vi "Old_Currentvstime.vi"() -> ()   [LabVIEW 2018]
uses:
  <userlib>/KE237.LLB/Keith 237 Operate/Standby.vi
  <vilib>/Utility/file.llb/Write To Spreadsheet File (string).vi
  <instrlib>/Keithley 24XX/Keithley 24XX.lvlib
  <vilib>/Analysis/NI_AALBase.lvlib
panel:
  in  "Autozero?":u16(ring)=2 items=["On", "Off", "Once"]
  in  "Measurement Speed (1 PLC)":dbl=1.0 format="%.2g"
  in  "Manual Range (Max I)":dbl=1.0
  in  "Enable Meas Auto Range":bool=TRUE
  in  "Source Mode":u16(ring) items=["Voltage", "Current"]
  in  "Measurement Gate Bias (V)":dbl=-0.85 format="%#.3g"
  in  "Initial Gate Bias (V)":dbl format="%#.3g"
  in  "Voltage Compliance Limit 237 (V)":dbl=10.0 format="%#.3f"
  in  "Current Compliance\nLimit 237 (A)":dbl=0.1 format="%#.3f"
  in  "Delay Gate (s)":dbl=60.0 format="%#.3g"
  in  "Keithley 237 GPIB address":string="17"
  in  "Wait Time Btwn Keithley Readings (ms)":i32=30
  out "Time Btwn Iterations (ms)":i32
  out "Total Elapsed Time (ms)":i32
  out "# Avgs":i32
  out "Current (A)":dbl format="%.2e"
  in  "Total Measure Time (s)":dbl=60.0 format="%#.3g"
  in  "Drain Bias (V)":dbl=-0.6 format="%#.3g"
  in  "Current Compliance\nLimit (A)":dbl=0.5 format="%#.3e"
  in  "Keithley 2400\nVISA resource":refnum<visa-resource-name>="GPIB0::24::INSTR"
  in  "Active Area (cm^2)":dbl=0.0122 min=0.0 format="%#.4e"
  in  "ApproximateTime Step (ms)":dbl=300.0 format="%#.3g"
  in  "Show Current:":enum32{"Density (mA/cm^2)", "Absolute (A)"}(radio)=enum."Absolute (A)"
  in  "Current Offset":dbl format="%^#_3e"
  out "I-t Measurement\nBy M. Ziffer 7/3/2014":cluster{dbl[], dbl[]}(graph)={[-2.0, -1.95, -1.9, -1.85, -1.8, -1.75, -1.7, -1.65, -1.6, -1.55, -1.5, -1.45, -1.4, -1.35, -1.2999999999999998, -1.25, -1.2, -1.15, -1.1, -1.0499999999999998, -1.0, -0.95, -0.8999999999999999, -0.8499999999999999, -0.7999999999999998, -0.75, -0.7, -0.6499999999999999, -0.5999999999999999, -0.5499999999999998, -0.5, -0.44999999999999996, -0.3999999999999999, -0.34999999999999987, -0.2999999999999998, -0.25, -0.19999999999999996, -0.1499999999999999, -0.09999999999999987, -0.04999999999999982, 0.0, 0.050000000000000266, 0.10000000000000009, 0.1499999999999999, 0.20000000000000018, 0.25, 0.30000000000000027, 0.3500000000000001, 0.40000000000000036, 0.4500000000000002, 0.5, 0.5500000000000003, 0.6000000000000001, 0.6500000000000004, 0.7000000000000002, 0.75, 0.8000000000000003, 0.8500000000000001, 0.9000000000000004, 0.9500000000000002, 1.0, 1.0500000000000003, 1.1, 1.1500000000000004, 1.2000000000000002, 1.25, 1.3000000000000003, 1.35, 1.4000000000000004, 1.4500000000000002, 1.5, 1.5500000000000003, 1.6, 1.6500000000000004, 1.7000000000000002, 1.75, 1.8000000000000003, 1.85, 1.9000000000000004, 1.9500000000000002, 2.0, 1.95, 1.9, 1.85, 1.8, 1.75, 1.7, 1.65, 1.6, 1.55, 1.5, 1.45, 1.4, 1.35, 1.2999999999999998, 1.25, 1.2, 1.15, 1.1, 1.0499999999999998, 1.0, 0.95, 0.8999999999999999, 0.8499999999999999, 0.7999999999999998, 0.75, 0.7, 0.6499999999999999, 0.5999999999999999, 0.5499999999999998, 0.5, 0.44999999999999996, 0.3999999999999999, 0.34999999999999987, 0.2999999999999998, 0.25, 0.19999999999999996, 0.1499999999999999, 0.09999999999999987, 0.04999999999999982, 0.0, -0.050000000000000266, -0.10000000000000009, -0.1499999999999999, -0.20000000000000018, -0.25, -0.30000000000000027, -0.3500000000000001, -0.40000000000000036, -0.4500000000000002, -0.5, -0.5500000000000003, -0.6000000000000001, -0.6500000000000004, -0.7000000000000002, -0.75, -0.8000000000000003, -0.8500000000000001, -0.9000000000000004, -0.9500000000000002, -1.0, -1.0500000000000003, -1.1, -1.1500000000000004, -1.2000000000000002, -1.25, -1.3000000000000003, -1.35, -1.4000000000000004, -1.4500000000000002, -1.5, -1.5500000000000003, -1.6, -1.6500000000000004, -1.7000000000000002, -1.75, -1.8000000000000003, -1.85, -1.9000000000000004, -1.9500000000000002, -2.0], [-0.9617289445307117, -0.9618513744908972, -0.9601574911889584, -0.9603488957746004, -0.9598860982876659, -0.9595594700613103, -0.9590290885663679, -0.9586886097902229, -0.9580144940757807, -0.9570474587019399, -0.9571418538143588, -0.9562287187728303, -0.9551771894828052, -0.9535572870291384, -0.9535421571112963, -0.9533114258642045, -0.9520938012261039, -0.9513117179729429, -0.9508812384355169, -0.9504840780921618, -0.9504173840793213, -0.9482281628421478, -0.9464640811713977, -0.9453356785488072, -0.9439408336230415, -0.9428695575652444, -0.9416178906119992, -0.9396031084275935, -0.9378375248899987, -0.9354517815949719, -0.9324159524550173, -0.928767917889437, -0.9245502864168607, -0.9203528467096396, -0.9146985405384399, -0.908595454304189, -0.9012966039381313, -0.8917361646028689, -0.8808115851751085, -0.8684870433493713, -0.853007079283089, -0.8360736418594031, -0.8154860511533626, -0.7920970894092216, -0.7641180332150388, -0.7294003786125389, -0.6854183749419586, -0.6263231964633708, -0.5399961516707377, -0.4044042921440459, -0.19129744134883978, 0.11936942255465804, 0.5420583260977958, 1.0996962734707192, 1.8318907919106253, 2.7834859177196174, 3.9948214605959804, 5.494887344369723, 7.293988211209965, 9.39251059714275, 11.765998658717283, 14.371720946722268, 17.153138293174568, 20.070768287470067, 23.082285540692517, 26.15604905590766, 29.26009131920428, 32.38734131897913, 35.54092126952808, 38.70923397757575, 41.89103456238207, 45.09512285116253, 48.318234786641504, 51.57411300669423, 54.84161623237131, 58.130390342544004, 61.4596508891188, 64.79419021952893, 68.17503711098149, 71.57587551887687, 75.0023346626475, 71.8977923333163, 68.72637799211101, 65.51757272894447, 62.2950059155054, 59.076872390492845, 55.84672949319313, 52.615591470047114, 49.383497814590335, 46.15858586388574, 42.93308596012382, 39.714879010509975, 36.494540522470736, 33.276879251143754, 30.087779593472593, 26.903443634933772, 23.758388169345494, 20.669969771208738, 17.671195580039395, 14.804861569698371, 12.12778391916459, 9.68736655227705, 7.528128139792144, 5.673530623057721, 4.128839936603901, 2.8787577310032053, 1.895544581260216, 1.1383875896205915, 0.5622048852612092, 0.12746496878202787, -0.18928305409978952, -0.4042961076690051, -0.5411369085387429, -0.6286316214282486, -0.6871327837574404, -0.7298882072135505, -0.7640718647157413, -0.7921132761963248, -0.8155779431543743, -0.8358809022810104, -0.8523300154596555, -0.8668520109778625, -0.8802307520791266, -0.8907705198464766, -0.8998007445608903, -0.9078572589377096, -0.9150023626386364, -0.9215738644543149, -0.925261336930741, -0.9288795566582202, -0.9332418679701618, -0.9352489739462505, -0.9376688708058178, -0.9394550911063516, -0.9405290371496502, -0.9430050037047499, -0.9440335043698243, -0.9453382929096107, -0.9473152502994113, -0.9474565926568992, -0.9494901203645137, -0.94896546821346, -0.9503187058651598, -0.9511280452203158, -0.9523093469306558, -0.9532668704811476, -0.9541692143312739, -0.9545545822386634, -0.955485183435348, -0.9561708134622656, -0.956805602515258, -0.9577699122788996, -0.9578049002139094, -0.9580356870856992, -0.958780001168953, -0.9592832934359943, -0.9588639388381576, -0.959203916992021, -0.9603773199952523, -0.9611007191920772, -0.9623172869609168]}
  in  "First bias settle (ms)":dbl=2000.0 format="%#.2f"
  out "Outputfile":path
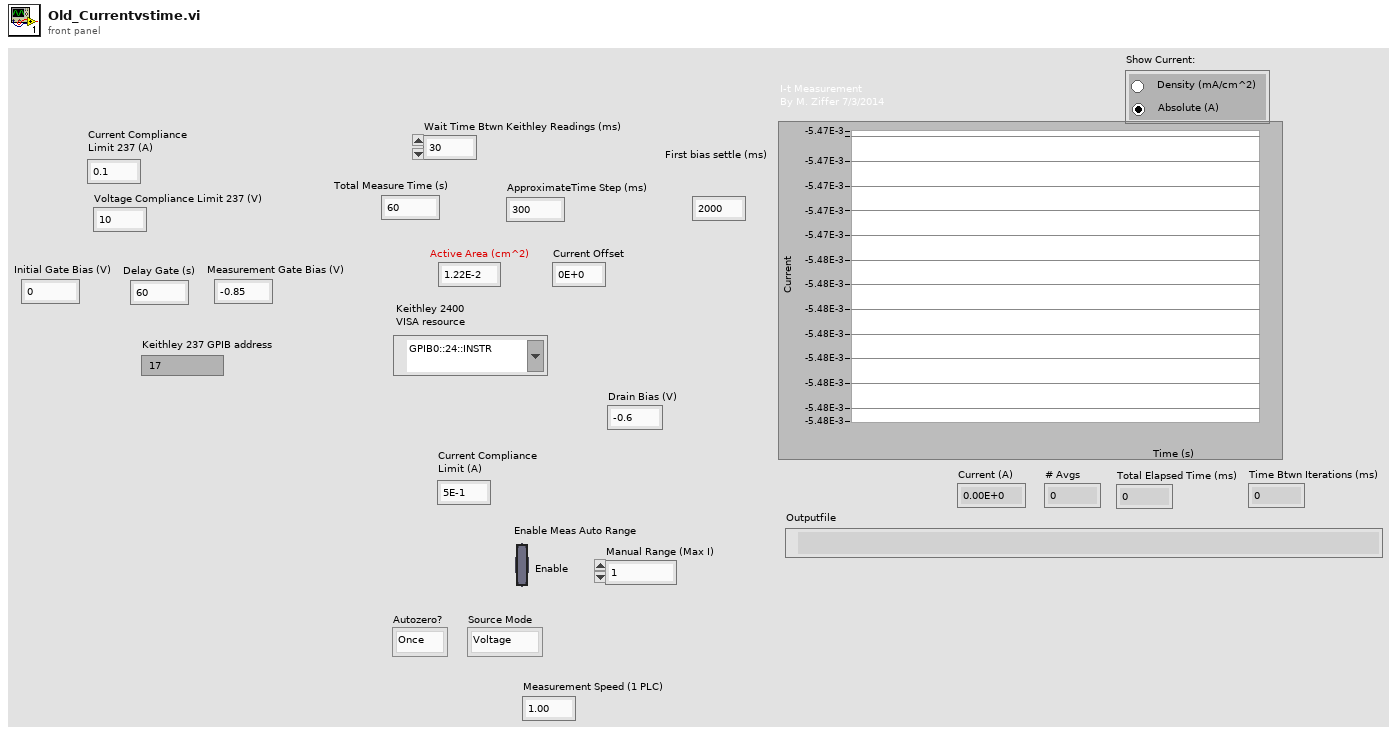
[diagram p1: front panel]
types:
  T1 = cluster{"error":bool, "code":i32, "source":string}
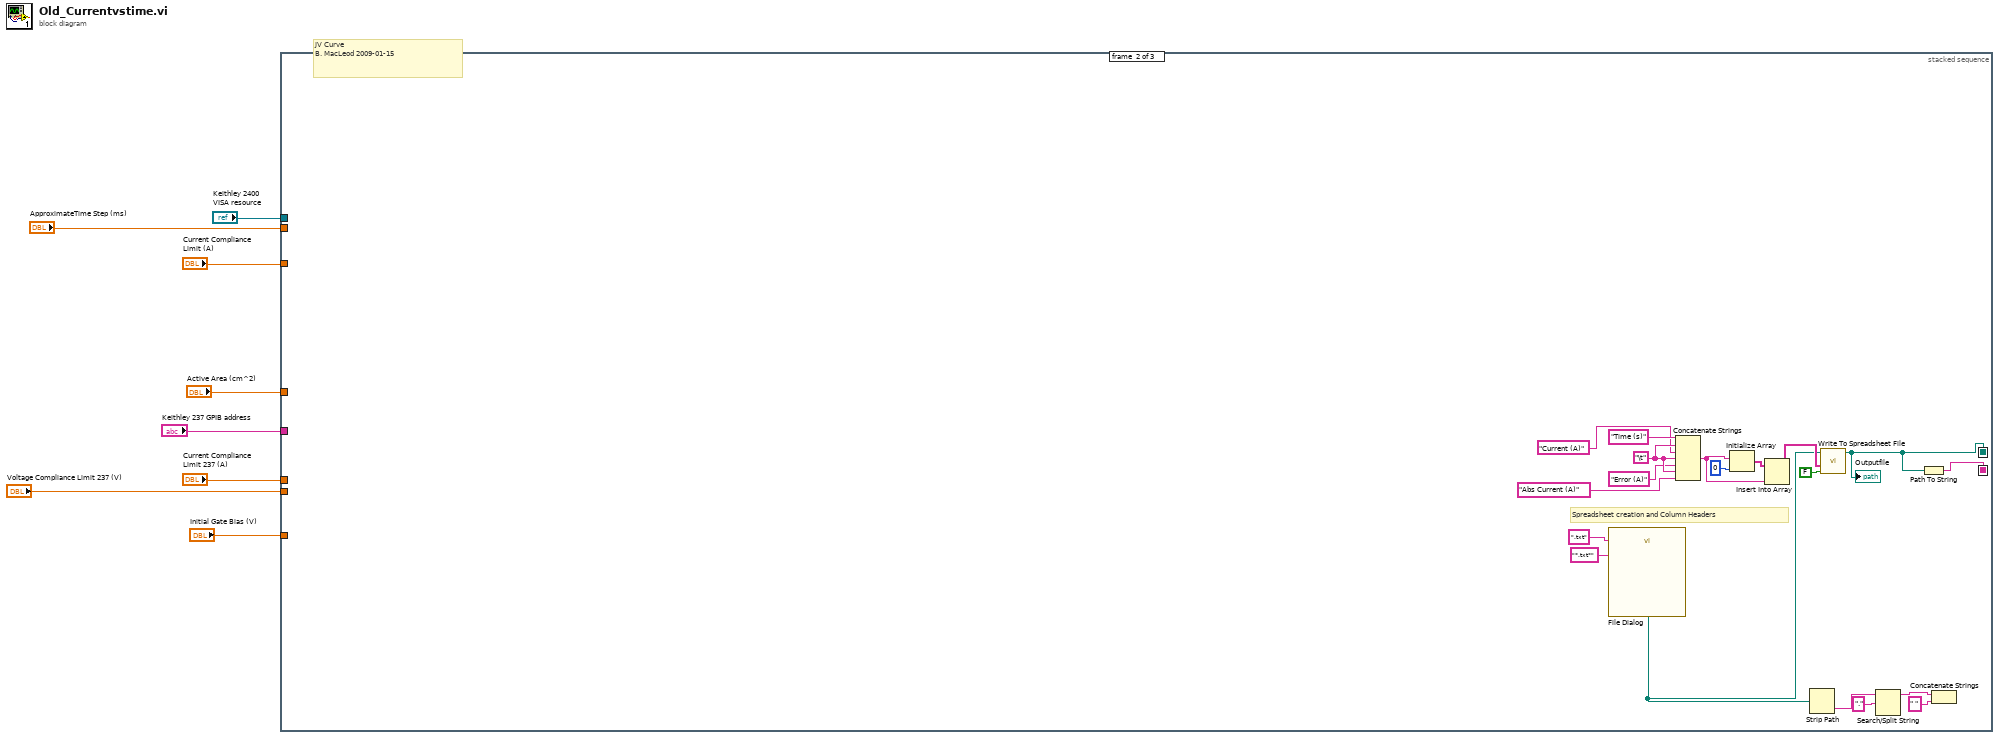
[diagram p0: block diagram]
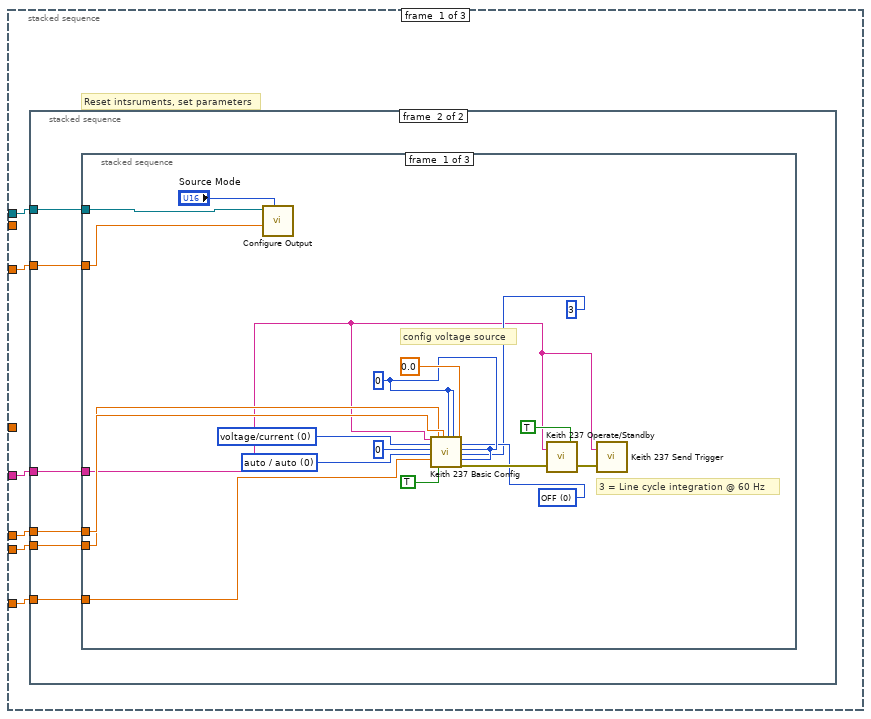
[diagram p2: hidden frame]
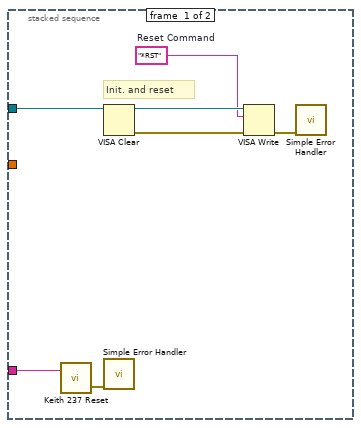
[diagram p3: hidden frame]
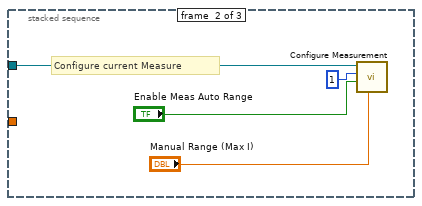
[diagram p4: hidden frame]
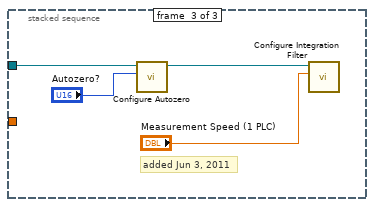
[diagram p5: hidden frame]
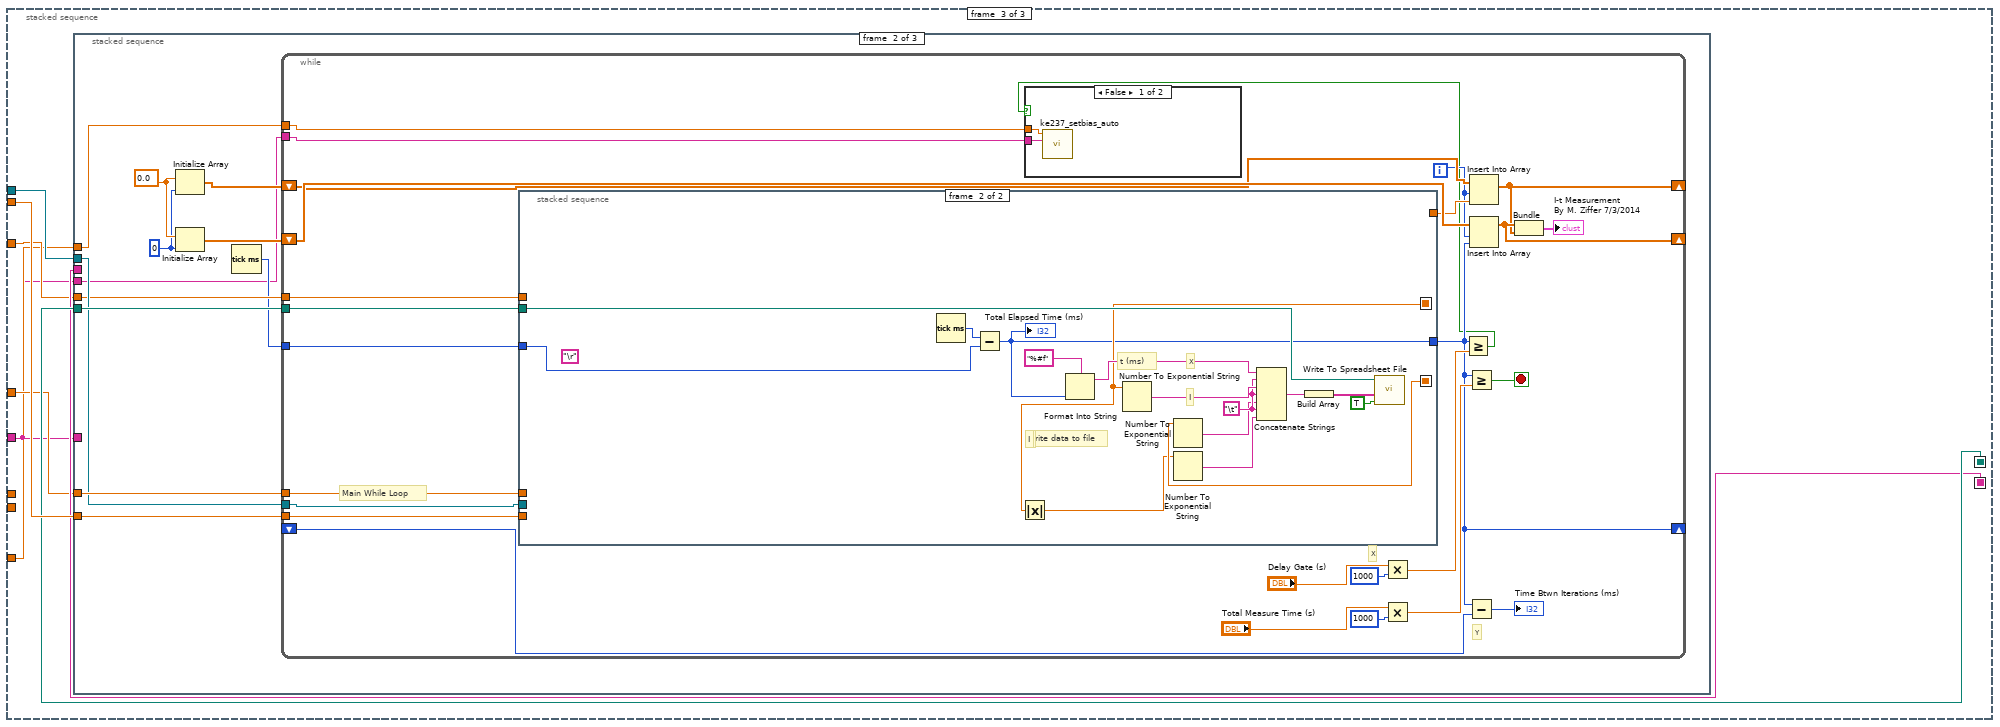
[diagram p6: hidden frame]
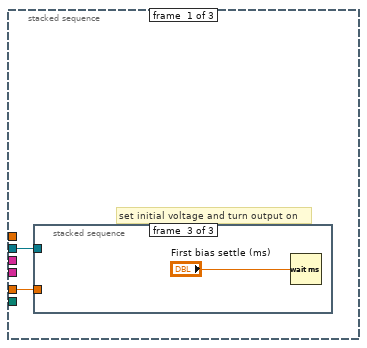
[diagram p7: hidden frame]
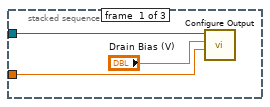
[diagram p8: hidden frame]
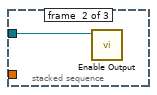
[diagram p9: hidden frame]
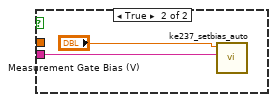
[diagram p10: hidden frame]
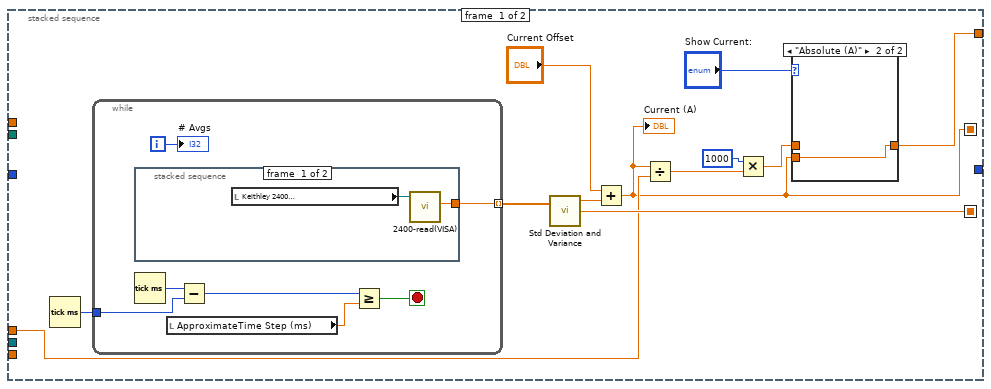
[diagram p11: hidden frame]
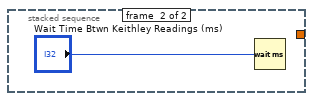
[diagram p12: hidden frame]
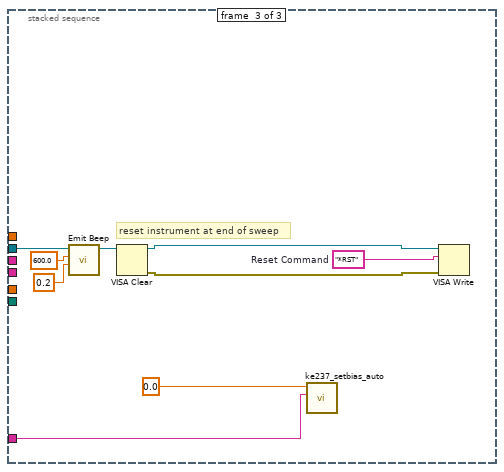
[diagram p14: hidden frame]
diagram:
  # "JV Curve\nB. MacLeod 2009-01-15"
  n1 = stacked-sequence {
    seq-local: [_ w71 _] -> [_ _ w79]
    seq-local: [_ w70 _] -> [_ _ w78]
    tunnel: "ApproximateTime Step (ms)" -> [_ _ w80]
    tunnel: "Active Area (cm^2)" -> [_ _ w77]
    tunnel: "Keithley 2400\nVISA resource" -> [w13 _ w75]
    tunnel: "Current Compliance\nLimit (A)" -> [w14 _ w76]
    tunnel: "Keithley 237 GPIB address" -> [w12 _ w73]
    tunnel: "Voltage Compliance Limit 237 (V)" -> [w10 _ _]
    tunnel: "Current Compliance\nLimit 237 (A)" -> [w11 _ _]
    tunnel: "Initial Gate Bias (V)" -> [w9 _ w74]
    frame #0 {
      # "Reset intsruments, set parameters"
      n2 = stacked-sequence {
        tunnel: w13 -> [w21 w26]
        tunnel: w14 -> [_ w27]
        tunnel: w12 -> [w15 w25]
        tunnel: w11 -> [_ w24]
        tunnel: w10 -> [_ w23]
        tunnel: w9 -> [_ w22]
        frame #0 {
          w19 = "*RST"  # Reset Command
          # "Init. and reset"
          n3 = call <userlib>:"Keith 237 Reset.vi"("GPIB address"=w15) -> ("error out"=w16:T1)  [unwired: 1 in]
          n4 = VISA Clear(VISA resource name=w21) -> (VISA resource name out=w20:refnum<visa-resource-name>, error out=w18:errorcluster)  [unwired: 1 in]
          n5 = call <vilib>:"Simple Error Handler.vi"("error in (no error)"=w16) -> ()  [unwired: 1 in, 8 out]
          n6 = VISA Write(VISA resource name=w20, write buffer=w19, error in (no error)=w18) -> (error out=w17:errorcluster)  [unwired: 2 out]
          n7 = call <vilib>:"Simple Error Handler.vi"("error in (no error)"=w17) -> ()  [unwired: 1 in, 8 out]
        }
        frame #1 {
          n8 = stacked-sequence {
            tunnel: w26 -> [w45 w48 w52]
            tunnel: w27 -> [w44 _ _]
            tunnel: w25 -> [w28 _ _]
            tunnel: w24 -> [w31 _ _]
            tunnel: w23 -> [w30 _ _]
            tunnel: w22 -> [w29 _ _]
            frame #0 {
              w33 = u16 0 items=["OFF", "ON"] ("default delay (on:1)")
              w34 = u16 0 items=["auto / auto", "1 nA / 1.1 V", "10 nA / 11 V", "100 nA / 110 V", "0.001 mA / 1100 V", "0.01 mA / 1100 V", "0.1 mA / 1100 V", "1 mA / 1100 V", "10 mA / 1100 V", "100 mA / 1100 V"] ("source range\nI source / V source (auto:0)")
              w35 = u16 0 items=["voltage/current", "current/voltage"] ("source/measure (V/I:0)")
              w37 = u16 0
              # "3 = Line cycle integration @ 60 Hz"
              # "config voltage source"
              n9 = call <instrlib>:"Configure Output.vi"("Source Mode  (0: Voltage)"="Source Mode", "Compliance  Level (0.1)"=w44, "VISA resource name"=w45) -> ()  [unwired: 3 in, 6 out]
              n10 = call <userlib>:"Keith 237 Basic Config.vi"("GPIB address"=w28, "source/measure (V/I:0)"=w35, "function (DC:0)"=u16 0, "source range\nI source / V source (auto:0)"=w34, "source level"=w29, "voltage \ncompliance level"=w30, "1100 V range (disabled:F)"=TRUE, "current \ncompliance level"=w31, "compliance/\nmeasurement range (auto:0)"=w37, "suppression (off:0)"=w37, "DC delay (sec)"=0.0, "default delay (on:1)"=w33, "filter (disabled:0)"=w37, "integration time (medium:1)"=u16 3, "sense (local:0)"=w37) -> ("error out"=w42:T1)  [unwired: 4 in]
              n11 = call "Keith 237 Operate/Standby.vi"("source"=TRUE, "error in"=w42, "GPIB address"=w28) -> ("error out"=w40:T1)
              n12 = call <userlib>:"Keith 237 Send Trigger.vi"("GPIB address"=w28, "error in"=w40) -> ()  [unwired: 1 out]
            }
            frame #1 {
              # "Configure current Measure"
              n13 = call <instrlib>:"Configure Measurement.vi"("Manual Range (1.0)"="Manual Range (Max I)", "Enable Auto Range (T:Enable)"="Enable Meas Auto Range", "Function (0: Volts)"=1, "VISA resource name"=w48) -> ()  [unwired: 1 in, 7 out]
            }
            frame #2 {
              # "added Jun 3, 2011"
              n14 = call <instrlib>:"Configure Autozero.vi"("Autozero  (0: On)"="Autozero?", "VISA resource name"=w52) -> ("VISA resource name out"=w51:refnum<visa-resource-name>)  [unwired: 1 in, 8 out]
              n15 = call <instrlib>:"Configure Integration Filter.vi"("Measurement Speed (1 PLC)"="Measurement Speed (1 PLC)", "VISA resource name"=w51) -> ()  [unwired: 8 in, 2 out]
            }
          }
        }
      }
    }
    frame #1 {
      w62 = "\t"
      # "Spreadsheet creation and Column Headers"
      n16 = call "File Dialog"("default name"=".txt", "pattern (all files)"="*.txt*") -> ("selected path"=w59:path)  [unwired: 5 in, 8 out]
      n17 = Concatenate Strings("Time (s)", w62, "Current (A)", w62, "Error (A)", w62, "Abs Current (A)" ("string")) -> (w67:string)
      n18 = Initialize Array(w67, 0 ("dimension size")) -> (w66:string[])
      n19 = Insert Into Array(array=w66, new element=w67) -> (w69:string[])  [unwired: 1 in]
      n20 = Strip Path(path=w59) -> (name=w58:string)  [unwired: 1 out]
      n21 = call-poly <vilib>:"Write To Spreadsheet File.vi"("append to file? (new file:F)"=FALSE, "1D data"=w69, "file path (dialog if empty)"=w59) -> ("new file path (Not A Path if cancelled)"=w71:path)  [unwired: 3 in, 2 out]
      "Outputfile" <- w71
      n22 = Search/Split String(string=w58, search string/char (-)=".") -> (substring before match=w61:string)  [unwired: 3 out]
      n23 = Path To String(path=w71) -> (string=w70:string)
      n24 = Concatenate Strings(w61, " " ("string")) -> ()  [unwired: 1 out]
    }
    frame #2 {
      n25 = stacked-sequence {
        tunnel: w80 -> [_ w91 _]
        tunnel: w79 -> [_ w99 _]
        tunnel: w78 -> [_ _ _]
        tunnel: w77 -> [_ w94 _]
        tunnel: w76 -> [w82 w92 _]
        tunnel: w75 -> [w81 w93 w175]
        tunnel: w73 -> [_ w89 _]
        tunnel: w74 -> [_ w88 _]
        tunnel: w73 -> [_ _ w170]
        frame #0 {
          # "set initial voltage and turn output on"
          n26 = stacked-sequence {
            tunnel: w81 -> [w84 w86 _]
            tunnel: w82 -> [w85 _ _]
            frame #0 {
              n27 = call <instrlib>:"Configure Output.vi"("Compliance  Level (0.1)"=w85, "Output Level (0)"="Drain Bias (V)", "VISA resource name"=w84) -> ()  [unwired: 3 in, 6 out]
            }
            frame #1 {
              n28 = call <instrlib>:"Enable Output.vi"("VISA resource name"=w86) -> ()  [unwired: 2 in, 9 out]
            }
            frame #2 {
              n29 = Wait (ms)(milliseconds to wait="First bias settle (ms)") -> ()  [unwired: 1 out]
            }
          }
        }
        frame #1 {
          w95 = 0
          w96 = 0.0
          n30 = Initialize Array(w96, w95) -> (w97:dbl[])
          n31 = Initialize Array(w96, w95) -> (w98:dbl[])
          n32 = Tick Count (ms)() -> (millisecond timer value=w90:u32)
          n33 = while {
            shift-left: w97 -> [w122]
            shift-right: [w116] -> _
            shift-left: w98 -> [w123]
            shift-right: [w118] -> _
            tunnel: w99 -> [w124]
            tunnel: w94 -> [w121]
            tunnel: w93 -> [w120]
            tunnel: w92 -> [w119]
            tunnel: w91 -> [w114]
            tunnel: w90 -> [w107]
            shift-right: [w103] -> _
            shift-left: _ -> [w112]
            tunnel: w89 -> [w102]
            tunnel: w88 -> [w101]
            i -> [w115]
            stop <- w113 stop-if-true
            # "Main While Loop"
            # "X"
            # "Y"
            n34 = stacked-sequence {
              seq-local: [w140 _] -> [_ w160]
              seq-local: [w131 _] -> [_ w158]
              tunnel: [w136 _] -> w117
              tunnel: w124 -> [_ w165]
              tunnel: w121 -> [w134 _]
              tunnel: w120 -> [_ _]
              tunnel: w119 -> [_ _]
              tunnel: w114 -> [_ _]
              tunnel: w107 -> [_ w155]
              tunnel: [_ w154] -> w103
              frame #0 {
                n35 = Tick Count (ms)() -> (millisecond timer value=w130:u32)
                n36 = while {
                  tunnel: [w148] -> w141 mode=indexing
                  tunnel: w130 -> [w146]
                  i -> [w147]
                  stop <- w144 stop-if-true
                  n37 = stacked-sequence {
                    tunnel: [w149 _] -> w148
                    frame #0 {
                      n38 = local read "Keithley 2400\nVISA resource"() -> (w150:refnum<visa-resource-name>)
                      n39 = call "2400-read(VISA).vi"("2400 VISA ID"=w150) -> ("Current"=w149:dbl)  [unwired: 6 out]
                    }
                    frame #1 {
                      n40 = Wait (ms)(milliseconds to wait="Wait Time Btwn Keithley Readings (ms)") -> ()  [unwired: 1 out]
                    }
                  }
                  n41 = Tick Count (ms)() -> (millisecond timer value=w143:u32)
                  n42 = local read "ApproximateTime Step (ms)"() -> (w142:dbl)
                  n43 = Subtract(x=w143, y=w146) -> (x-y=w145:u32)
                  n44 = Greater Or Equal?(x=w145, y=w142) -> (x >= y?=w144:bool)
                  "# Avgs" <- w147
                }
                n45 = call <vilib>:"Std Deviation and Variance.vi"("X"=w141) -> ("mean"=w133:dbl, "standard deviation"=w140:dbl)  [unwired: 1 in, 1 out]
                n46 = Add(x="Current Offset", y=w133) -> (x+y=w131:dbl)
                "Current (A)" <- w131
                n47 = Divide(x=w131, y=w134) -> (x/y=w139:dbl)
                n48 = Multiply(x=1000, y=w139) -> (x*y=w135:dbl)
                n49 = case shown="\"Absolute (A)\"" "Show Current:" {
                  tunnel: [w152 w153] -> w136
                  tunnel: w135 -> [w152 _]
                  tunnel: w131 -> [_ w153]
                  frame "Density (mA/cm^2)", Default {
                  }
                  frame "Absolute (A)" {
                  }
                }
              }
              frame #1 {
                (unwired) "\r"
                w162 = "\t"
                # "I"
                # "I"
                # "J"
                # "t (ms)"
                # "write data to file"
                # "X"
                n50 = Tick Count (ms)() -> (millisecond timer value=w156:u32)
                n51 = Subtract(x=w156, y=w155) -> (x-y=w154:u32)
                "Total Elapsed Time (ms)" <- w154
                n52 = Absolute Value(x=w158) -> (abs(x)=w159:dbl)
                n53 = Format Into String(format string="%#f", w154) -> (resulting string=w168:string)  [unwired: 2 in, 1 out]
                n54 = Number To Exponential String(number=w158) -> (E-format string=w167:string)  [unwired: 3 out]
                n55 = Number To Exponential String(number=w160) -> (E-format string=w161:string)  [unwired: 3 out]
                n56 = Number To Exponential String(number=w159) -> (E-format string=w157:string)  [unwired: 3 out]
                n57 = Concatenate Strings(w168, w162, w167, w162, w161, w162, w157) -> (w166:string)
                n58 = Build Array(w166) -> (w164:string[])
                n59 = call-poly <vilib>:"Write To Spreadsheet File.vi"("append to file? (new file:F)"=TRUE, "1D data"=w164, "file path (dialog if empty)"=w165) -> ()  [unwired: 3 in, 3 out]
              }
            }
            n60 = Multiply(x="Delay Gate (s)", y=1000) -> (x*y=w106:dbl)
            n61 = Multiply(x="Total Measure Time (s)", y=1000) -> (x*y=w108:dbl)
            n62 = Greater Or Equal?(x=w103, y=w106) -> (x >= y?=w100:bool)
            n63 = case shown="False" w100 {
              tunnel: w102 -> [w127 w129]
              tunnel: w101 -> [w126 _]
              frame False {
                n64 = call "ke237_setbias_auto.vi"("GPIB address"=w127, "source level"=w126) -> ()  [unwired: 10 in]
              }
              frame True {
                n65 = call "ke237_setbias_auto.vi"("GPIB address"=w129, "source level"="Measurement Gate Bias (V)") -> ()  [unwired: 10 in]
              }
            }
            n66 = Greater Or Equal?(x=w103, y=w108) -> (x >= y?=w113:bool)
            n67 = Subtract(x=w103, y=w112) -> (x-y=→"Time Btwn Iterations (ms)":u32)
            n68 = Insert Into Array(array=w122, index=w115, new element=w117) -> (w116:dbl[])
            n69 = Insert Into Array(array=w123, index=w115, new element=w103) -> (w118:dbl[])
            n70 = Bundle(w118, w116) -> (→"I-t Measurement\nBy M. Ziffer 7/3/2014":cluster{dbl[], dbl[]})  [unwired: 1 out]
          }
        }
        frame #2 {
          w177 = "*RST"  # Reset Command
          # "reset instrument at end of sweep"
          n71 = call <instrlib>:"Emit Beep.vi"("Beep Duration (.25 s)"=0.2, "Beep Frequency (300)"=600.0, "VISA resource name"=w175) -> ("VISA resource name out"=w174:refnum<visa-resource-name>)  [unwired: 7 in, 1 out]
          n72 = VISA Clear(VISA resource name=w174) -> (VISA resource name out=w178:refnum<visa-resource-name>, error out=w176:errorcluster)  [unwired: 1 in]
          n73 = call "ke237_setbias_auto.vi"("GPIB address"=w170, "source level"=0.0) -> ()  [unwired: 10 in]
          n74 = VISA Write(VISA resource name=w178, write buffer=w177, error in (no error)=w176) -> ()  [unwired: 3 out]
        }
      }
    }
  }
